vi "coords_image_to_real_currentimage.vi"(1 "Position (pixels on image)":cluster{"X":dbl, "Y":dbl}, 4 "z (real coords)":dbl) -> (8 "Position (real coords)":cluster{dbl, dbl, "Z":dbl})   [LabVIEW 2010]
uses:
  red_tweezers_globals_INTERNAL.vi
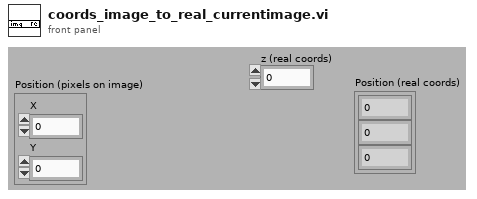
[diagram p1: front panel]
types:
  T1 = cluster{"Global ROI[0]":i32, "Global ROI[1]":i32}
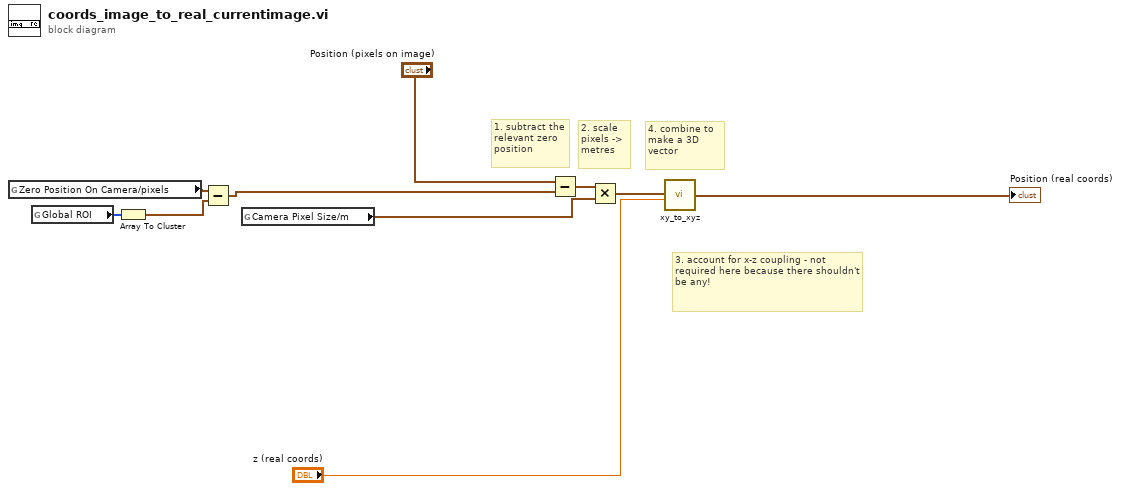
[diagram p0: block diagram]
diagram:
  # "3. account for x-z coupling - not required here because there shouldn't be any!"
  # "4. combine to make a 3D vector"
  # "2. scale pixels -> metres"
  # "1. subtract the relevant zero position"
  n1 = global read "red_tweezers_globals_INTERNAL.vi" "Zero Position On Camera/pixels"() -> (w3:cluster{"X":dbl, "Y":dbl})
  n2 = global read "red_tweezers_globals_INTERNAL.vi" "Global ROI"() -> (w4:i32[])
  n3 = Array To Cluster(array=w4) -> (cluster=w2:T1)
  n4 = Subtract(x=w3, y=w2) -> (x-y=w1:cluster{dbl, dbl})
  n5 = global read "red_tweezers_globals_INTERNAL.vi" "Camera Pixel Size/m"() -> (w10:cluster{dbl, dbl})
  n6 = Subtract(x="Position (pixels on image)", y=w1) -> (x-y=w5:cluster{dbl, dbl})
  n7 = Multiply(x=w5, y=w10) -> (x*y=w6:cluster{dbl, dbl})
  n8 = call "xy_to_xyz.vi"("z"="z (real coords)", "Position (2D)"=w6) -> ("Position (3D)"=→"Position (real coords)":cluster{dbl, dbl, dbl})  [unwired: 2 in]
